vi "Remove.vi"(8 "error in (no error)":errorcluster, 10 "Module ID":i32=-1, 11 "CloneRegRef":refnum<data-value>) -> (0 "error out":errorcluster, 2 "Found?":bool, 3 "CloneRegRef":refnum<data-value>)   [LabVIEW 2018, in "ModuleAdmin.lvlib" / "CloneRegistration.lvclass"]
uses:
  CloneRegistration.lvclass
  CloneRegistration.lvclass/CloneRegistration.ctl
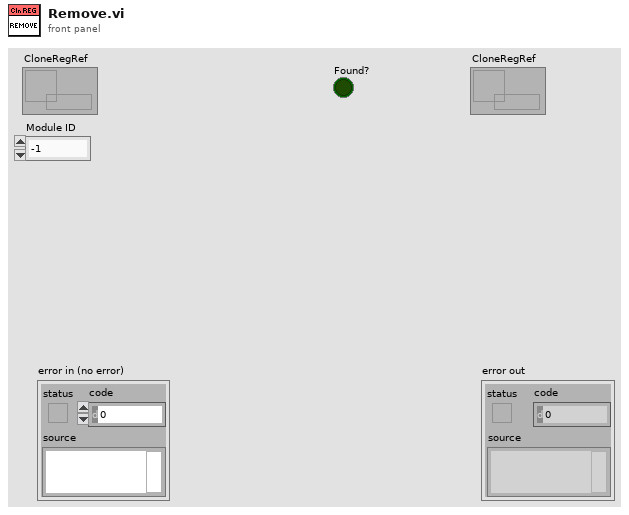
[diagram p1: front panel]
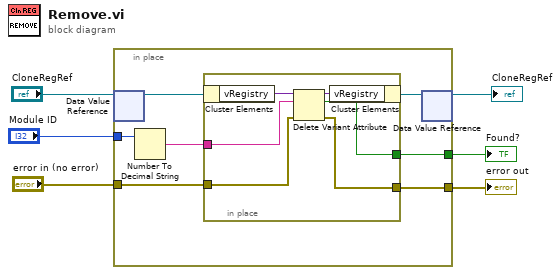
[diagram p0: block diagram]
diagram:
  n1 = in-place {
    in-place-border: "Module ID" -> [w13]
    in-place-border: "error in (no error)" -> [w11]
    in-place-border: [w10] -> w4
    in-place-border: [w9] -> w3
    n2 = in-place-dvr #1("CloneRegRef") -> (w8:refnum<class "CloneRegistration.lvclass">)  [unwired: 1 out]
    n3 = Number To Decimal String(number=w13) -> (decimal integer string=w12:string)  [unwired: 1 in]
    n4 = in-place {
      in-place-border: w12 -> [w18]
      in-place-border: w11 -> [w16]
      in-place-border: [w15] -> w10
      in-place-border: [w17] -> w9
      n5 = in-place-cluster #2(w8) -> ("vRegistry"=w19:variant)
      n6 = Delete Variant Attribute(4:w16, 6:w18, 7:w19) -> (0:w15:errorcluster, 2:w17:bool, 3:w14:variant)
      n7 = in-place-cluster #2("vRegistry"=w14) -> (w7:refnum<class "CloneRegistration.lvclass">)
    }
    n8 = in-place-dvr #1(w7) -> (→"CloneRegRef":refnum<data-value>)  [unwired: 1 out]
  }
  "error out" <- w4
  "Found?" <- w3
